vi "ReadWire.vi"(1 "reference":refnum<vi>) -> (0 "Wire":T5)   [LabVIEW 2013]
uses:
  <vilib>/Utility/miscctls.llb/LVBoundsTypeDef.ctl
  <vilib>/Utility/miscctls.llb/LVPositionTypeDef.ctl
  <vilib>/Utility/miscctls.llb/LVRectTypeDef.ctl
  <vilib>/Utility/miscctls.llb/LVBreakpointStatusEnum.ctl
panel:
  out "error out 22":errorcluster
  out "error out 21":errorcluster
  out "error out 20":errorcluster
  out "error out 19":errorcluster
  out "error out 18":errorcluster
  out "error out 17":errorcluster
  out "error out 16":errorcluster
  out "error out 15":errorcluster
  out "error out 14":errorcluster
  out "error out 13":errorcluster
  out "error out 12":errorcluster
  out "error out 11":errorcluster
  out "error out 10":errorcluster
  out "error out 9":errorcluster
  out "error out 8":errorcluster
  out "error out 7":errorcluster
  out "error out 6":errorcluster
  out "error out 5":errorcluster
  out "error out 4":errorcluster
  out "error out 3":errorcluster
  out "error out 2":errorcluster
  out "error out":errorcluster
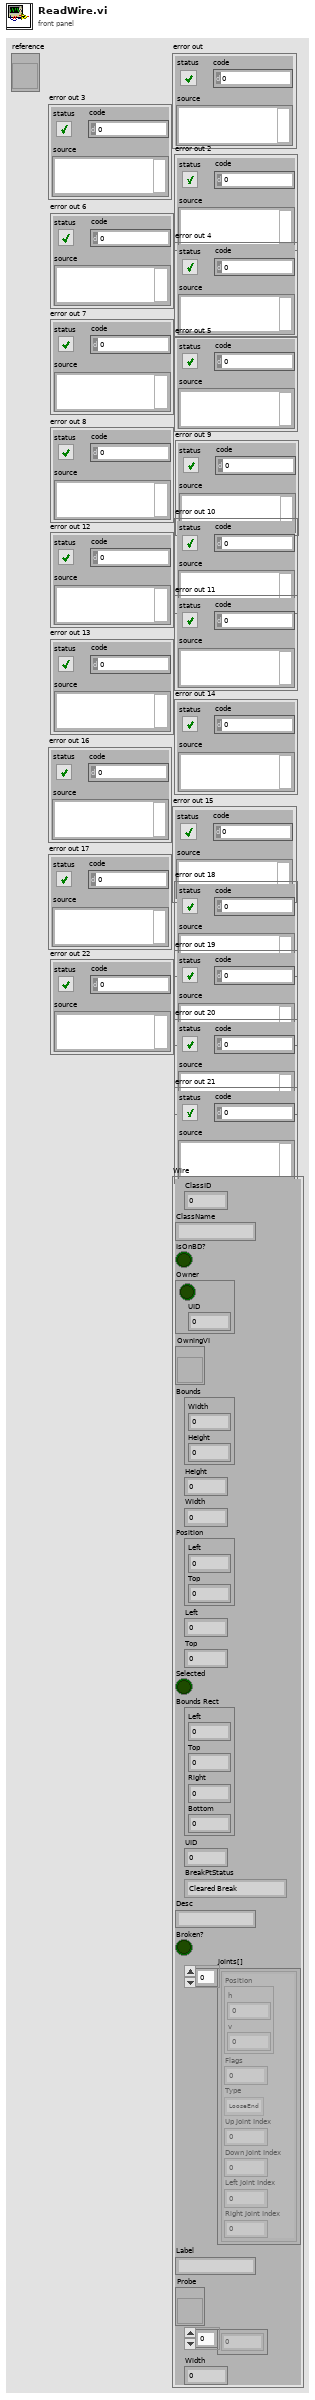
[diagram p1: front panel]
types:
  T1 = typedef "LVBoundsTypeDef.ctl" = cluster{"Width":u32, "Height":u32}
  T2 = typedef "LVPositionTypeDef.ctl" = cluster{"Left":i32, "Top":i32}
  T3 = typedef "LVRectTypeDef.ctl" = cluster{"Left":i16, "Top":i16, "Right":i16, "Bottom":i16}
  T4 = typedef "LVBreakpointStatusEnum.ctl" = enum8{"Cleared Break", "Enabled Break", "Disabled Break"}
  T5 = cluster{"ClassID":u32, "ClassName":string, "IsOnBD?":bool, "Owner":cluster{bool, "UID":i32}, "OwningVI":refnum<vi>, "Bounds":T1, "Height":u32, "Width":u32, "Position":T2, "Left":i32, "Top":i32, "Selected":bool, "Bounds Rect":T3, "UID":i32, "BreakPtStatus":T4, "Desc":string, "Broken?":bool, "Joints[]":cluster{"Position":cluster{"h":i16, "v":i16}, "Flags":i32, "Type":enum32{"LooseEnd", "Endpoint", "Bend", "Junction"}, "Up Joint Index":i16, "Down Joint Index":i16, "Left Joint Index":i16, "Right Joint Index":i16}[], "Label":string, "Probe":refnum<vi>, "Terms[]":i32[], "Width":u32}
  T6 = cluster{"Position":cluster{"h":i16, "v":i16}, "Flags":i32, "Type":enum32{"LooseEnd", "Endpoint", "Bend", "Junction"}, "Up Joint Index":i16, "Down Joint Index":i16, "Left Joint Index":i16, "Right Joint Index":i16}[]
  T7 = cluster{"ClassID":u32, "ClassName":string, "IsOnBD?":bool, "Cluster":cluster{bool, "UID":i32}, "OwningVI":refnum<vi>, "Bounds":T1, "Height":u32, "Width":u32, "Position":T2, "Left":i32, "Top":i32, "Selected":bool, "Bounds Rect":T3, "UID":i32, "BreakPtStatus":T4, "Desc":string, "Broken?":bool, "Joints[]":cluster{"Position":cluster{"h":i16, "v":i16}, "Flags":i32, "Type":enum32{"LooseEnd", "Endpoint", "Bend", "Junction"}, "Up Joint Index":i16, "Down Joint Index":i16, "Left Joint Index":i16, "Right Joint Index":i16}[], "Text":string, "Probe":refnum<vi>, i32[], "Width":u32}
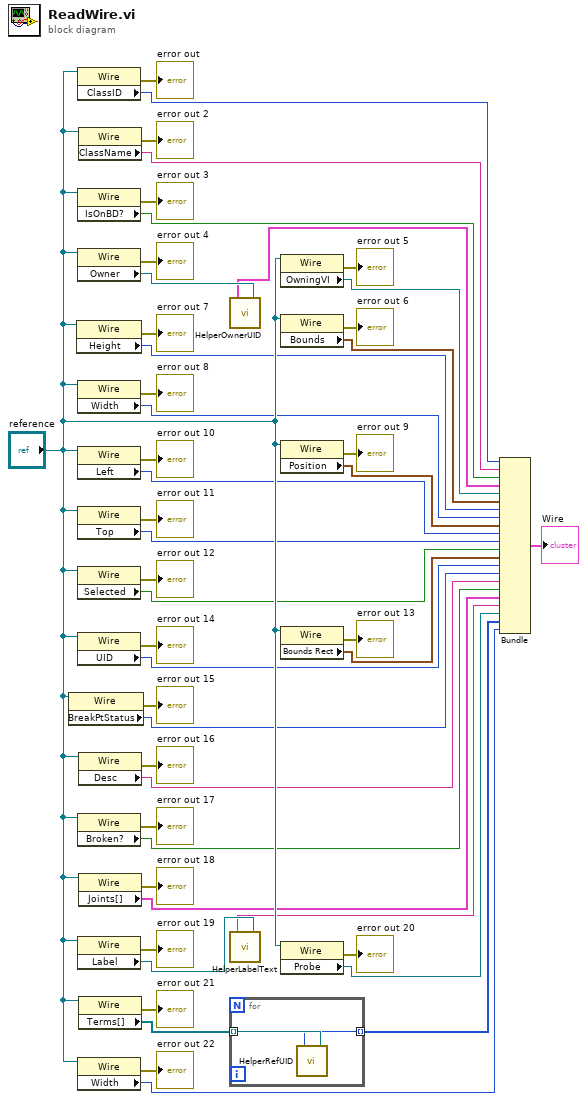
[diagram p0: block diagram]
diagram:
  n1 = property class="Wire"(reference="reference") -> (error out=→"error out 15":errorcluster, "BreakPtStatus"=w18:T4)  [unwired: 1 in, 1 out]
  n2 = property class="Wire"(reference="reference") -> (error out=→"error out 7":errorcluster, "Height"=w34:u32)  [unwired: 1 in, 1 out]
  n3 = property class="Wire"(reference="reference") -> (error out=→"error out":errorcluster, "ClassID"=w47:u32)  [unwired: 1 in, 1 out]
  n4 = property class="Wire"(reference="reference") -> (error out=→"error out 3":errorcluster, "IsOnBD?"=w43:bool)  [unwired: 1 in, 1 out]
  n5 = property class="Wire"(reference="reference") -> (error out=→"error out 4":errorcluster, "Owner"=w41:refnum<vi>)  [unwired: 1 in, 1 out]
  n6 = property class="Wire"(reference="reference") -> (error out=→"error out 8":errorcluster, "Width"=w32:u32)  [unwired: 1 in, 1 out]
  n7 = property class="Wire"(reference="reference") -> (error out=→"error out 10":errorcluster, "Left"=w28:i32)  [unwired: 1 in, 1 out]
  n8 = property class="Wire"(reference="reference") -> (error out=→"error out 11":errorcluster, "Top"=w26:i32)  [unwired: 1 in, 1 out]
  n9 = property class="Wire"(reference="reference") -> (error out=→"error out 12":errorcluster, "Selected"=w24:bool)  [unwired: 1 in, 1 out]
  n10 = property class="Wire"(reference="reference") -> (error out=→"error out 14":errorcluster, "UID"=w20:i32)  [unwired: 1 in, 1 out]
  n11 = property class="Wire"(reference="reference") -> (error out=→"error out 17":errorcluster, "Broken?"=w14:bool)  [unwired: 1 in, 1 out]
  n12 = property class="Wire"(reference="reference") -> (error out=→"error out 19":errorcluster, "Label"=w10:refnum<vi>)  [unwired: 1 in, 1 out]
  n13 = property class="Wire"(reference="reference") -> (error out=→"error out 22":errorcluster, "Width"=w2:u32)  [unwired: 1 in, 1 out]
  n14 = property class="Wire"(reference="reference") -> (error out=→"error out 2":errorcluster, "ClassName"=w45:string)  [unwired: 1 in, 1 out]
  n15 = property class="Wire"(reference="reference") -> (error out=→"error out 16":errorcluster, "Desc"=w16:string)  [unwired: 1 in, 1 out]
  n16 = property class="Wire"(reference="reference") -> (error out=→"error out 18":errorcluster, "Joints[]"=w12:T6)  [unwired: 1 in, 1 out]
  n17 = property class="Wire"(reference="reference") -> (error out=→"error out 21":errorcluster, "Terms[]"=w5:refnum<vi>[])  [unwired: 1 in, 1 out]
  n18 = call "HelperOwnerUID.vi"("Generic in"=w41) -> ("Cluster"=w40:cluster{bool, "UID":i32})
  n19 = call "HelperLabelText.vi"("Text in"=w10) -> ("Text"=w9:string)
  n20 = for {
    tunnel: w5 -> [w51] mode=indexing
    tunnel: [w50] -> w4 mode=indexing
    n21 = call "HelperRefUID.vi"("Text in"=w51) -> ("UID"=w50:i32)
  }
  n22 = property class="Wire"(reference="reference") -> (error out=→"error out 5":errorcluster, "OwningVI"=w38:refnum<vi>)  [unwired: 1 in, 1 out]
  n23 = property class="Wire"(reference="reference") -> (error out=→"error out 6":errorcluster, "Bounds"=w36:T1)  [unwired: 1 in, 1 out]
  n24 = property class="Wire"(reference="reference") -> (error out=→"error out 9":errorcluster, "Position"=w30:T2)  [unwired: 1 in, 1 out]
  n25 = property class="Wire"(reference="reference") -> (error out=→"error out 13":errorcluster, "Bounds Rect"=w22:T3)  [unwired: 1 in, 1 out]
  n26 = property class="Wire"(reference="reference") -> (error out=→"error out 20":errorcluster, "Probe"=w7:refnum<vi>)  [unwired: 1 in, 1 out]
  n27 = Bundle("ClassID"=w47, "ClassName"=w45, "IsOnBD?"=w43, "Cluster"=w40, "OwningVI"=w38, "Bounds"=w36, "Height"=w34, "Width"=w32, "Position"=w30, "Left"=w28, "Top"=w26, "Selected"=w24, "Bounds Rect"=w22, "UID"=w20, "BreakPtStatus"=w18, "Desc"=w16, "Broken?"=w14, "Joints[]"=w12, "Text"=w9, "Probe"=w7, w4, "Width"=w2) -> (→"Wire":T7)  [unwired: 1 in]
